vi "SetRecordFocus2DListCtrl.vi"(10 "index":u16, 11 "multiple list in":refnum<vi>) -> (3 "multiple list out":refnum<vi>)   [LabVIEW 2018, in "Library-Ctrl.lvlib"]
uses:
  Library-Ctrl.lvlib
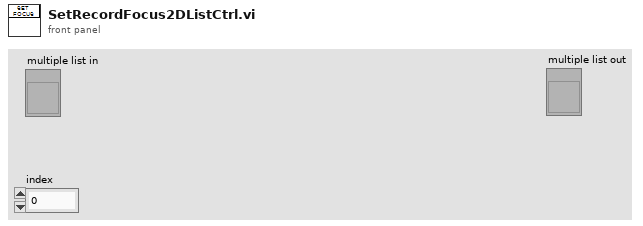
[diagram p1: front panel]
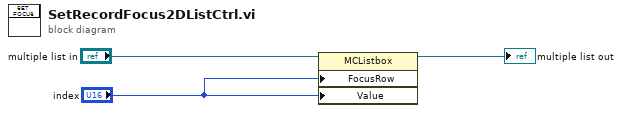
[diagram p0: block diagram]
diagram:
  n1 = property class="MCListbox"(reference="multiple list in", "FocusRow"="index", "Value"="index") -> (reference out=→"multiple list out":refnum<vi>)  [unwired: 1 in, 1 out]
